vi "GetAngles.vi"(11 "NewVal":path) -> (1 "Number of Rows":i32, 2 "Number of Angles":i32, 3 "Array":dbl[](array[numeric]))   [LabVIEW 2013]
panel:
  out "error out":errorcluster
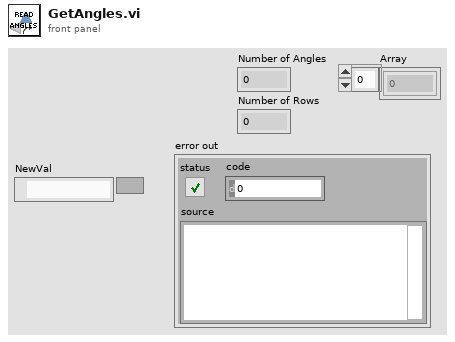
[diagram p1: front panel]
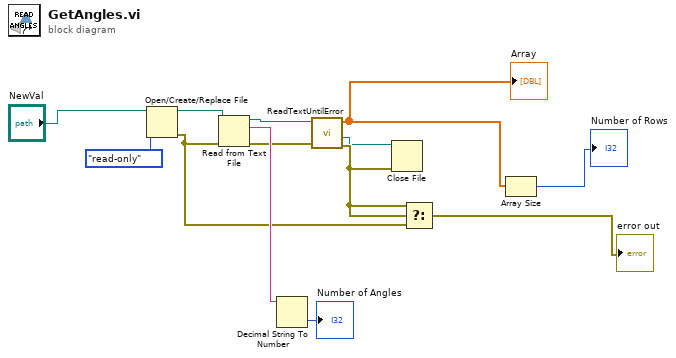
[diagram p0: block diagram]
diagram:
  n1 = Open/Create/Replace File(file path (use dialog)="NewVal", access (0:read/write)=enum16{"read/write", "read-only", "write-only"}."read-only") -> (refnum out=w11:refnum<file>, error out=w3:errorcluster)  [unwired: 4 in, 1 out]
  n2 = Read from Text File(file (use dialog)=w11, error in=w3) -> (refnum out=w10:refnum<file>, text=w9:string, error out=w4:errorcluster)  [unwired: 2 in, 1 out]
  n3 = Decimal String To Number(string=w9) -> (number=→"Number of Angles":i32)  [unwired: 2 in, 1 out]
  n4 = call "ReadTextUntilError.vi"("error in (no error)"=w4, "Byte Stream File in"=w10) -> ("error out"=w7:errorcluster, "refnum out"=w6:refnum<file>, "Array"=w1:dbl[])  [unwired: 7 in]
  "Array" <- w1
  n5 = Close File(refnum=w6, error in=w7) -> ()  [unwired: 2 out]
  n6 = Select(t=w7, s=w7, f=w3) -> (s? t:f=→"error out":errorcluster)
  n7 = Array Size(array=w1) -> (size(s)=→"Number of Rows":i32)
